vi "GetErrorBehavior.vi"(8 "error in (no error)":errorcluster, 11 "SMO in":refnum<class "SMO.lvclass">) -> (0 "error out":errorcluster, 2 "Shutdown on Unhandled Error":bool, 3 "SMO out":refnum<class "SMO.lvclass">)   [LabVIEW 2013, in "SMO.lvclass"]
uses:
  SMO.lvclass
  Support/Attribute.ErrorHandling/Attribute.ErrorHandling.lvclass
  SMO.lvclass/SMO.ctl
  Support/Attribute.ErrorHandling/Attribute.ErrorHandling.lvclass/Attribute.ErrorHandling.ctl
  ReftoDVR--SMO.vi
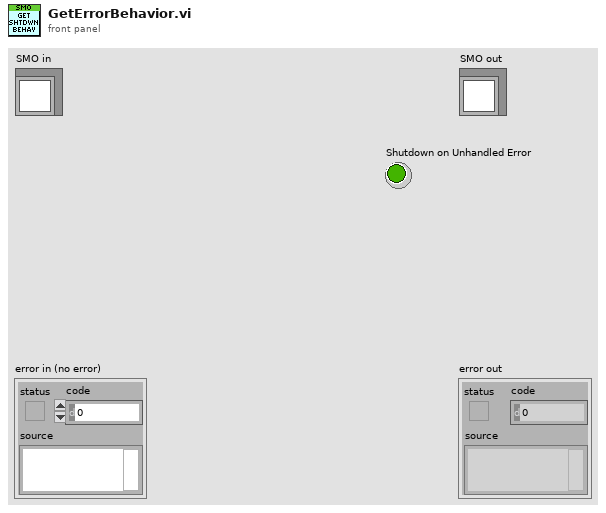
[diagram p1: front panel]
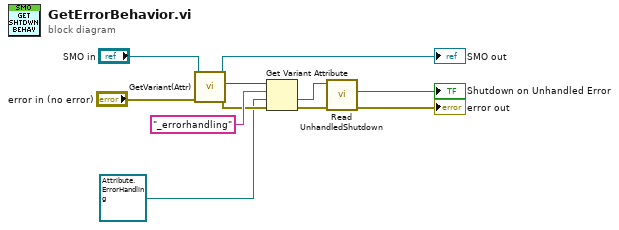
[diagram p0: block diagram]
diagram:
  n1 = call "GetVariant(Attr).vi"("error in (no error)"="error in (no error)", "SMO in"="SMO in") -> ("error out"=w9:errorcluster, "[Attributes]"=w11:variant, "SMO out"=→"SMO out":refnum<class "SMO.lvclass">)  [unwired: 7 in]
  n2 = Get Variant Attribute(Variant=w11, name="_errorhandling", default value (empty Variant)=refnum<class "Attribute.ErrorHandling.lvclass"> refnum ("Attribute.ErrorHandling.lvclass"), error in=w9) -> (value=w4:refnum<class "Attribute.ErrorHandling.lvclass">, error out=w3:errorcluster)  [unwired: 2 out]
  n3 = call "Read UnhandledShutdown.vi"("error in (no error)"=w3, "Attribute.StartupBehavior in"=w4) -> ("error out"=→"error out":errorcluster, "Shutdown on Unhandled Error"=→"Shutdown on Unhandled Error":bool)  [unwired: 7 in, 1 out]
